vi "GetTrigList.vi"(10 "List":u32) -> (2 "Trigger mode List":string)   [LabVIEW 2015]
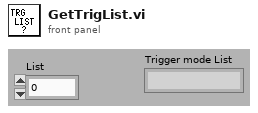
[diagram p1: front panel]
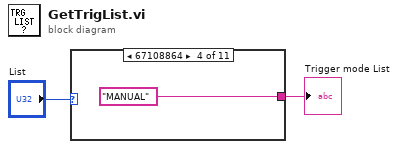
[diagram p0: block diagram]
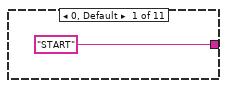
[diagram p2: hidden frame]
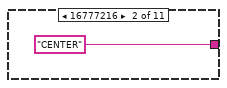
[diagram p3: hidden frame]
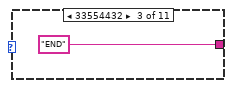
[diagram p4: hidden frame]
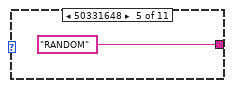
[diagram p5: hidden frame]
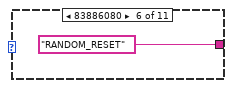
[diagram p6: hidden frame]
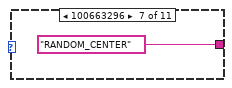
[diagram p7: hidden frame]
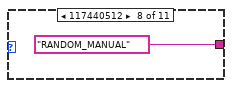
[diagram p8: hidden frame]
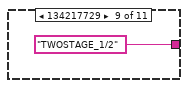
[diagram p9: hidden frame]
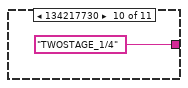
[diagram p10: hidden frame]
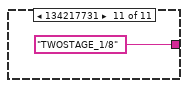
[diagram p11: hidden frame]
diagram:
  n1 = case shown="67108864" "List" {
    tunnel: ["START" "CENTER" "END" "MANUAL" "RANDOM" "RANDOM_RESET" "RANDOM_CENTER" "RANDOM_MANUAL" "TWOSTAGE_1/2" "TWOSTAGE_1/4" "TWOSTAGE_1/8"] -> w2
    frame 0, Default {
    }
    frame 16777216 {
    }
    frame 33554432 {
    }
    frame 67108864 {
    }
    frame 50331648 {
    }
    frame 83886080 {
    }
    frame 100663296 {
    }
    frame 117440512 {
    }
    frame 134217729 {
    }
    frame 134217730 {
    }
    frame 134217731 {
    }
  }
  "Trigger mode List" <- w2
